vi "WaveformToArrayOfDbl.vi"(11 "waveform":waveform(dbl)) -> (3 "Array":dbl[][](array[numeric]))   [LabVIEW 2013]
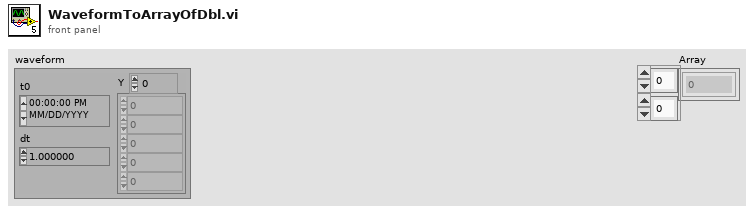
[diagram p1: front panel]
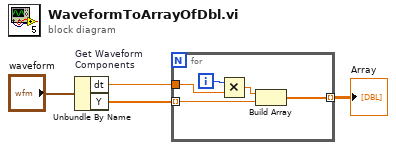
[diagram p0: block diagram]
diagram:
  n1 = Unbundle By Name "Get Waveform Components"("waveform") -> ("dt"=w3:dbl, "Y"=w2:dbl[])
  n2 = for {
    tunnel: w3 -> [w9]
    tunnel: w2 -> [w7] mode=indexing
    tunnel: [w5] -> w1 mode=indexing
    i -> [w8]
    n3 = Multiply(x=w8, y=w9) -> (x*y=w6:dbl)
    n4 = Build Array "Build Array"(w6, w7) -> (w5:dbl[])
  }
  "Array" <- w1
